vi "GraphSetting Conv Log.vi"(11 "XScale.Mapping Mode":u8) -> (3 "ログ?":bool)   [LabVIEW 2016]
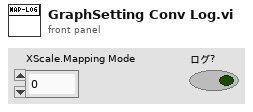
[diagram p1: front panel]
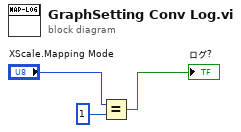
[diagram p0: block diagram]
diagram:
  n1 = Equal?(x="XScale.Mapping Mode", y=u8 1) -> (x = y?=→"ログ?":bool)
